vi "ESW (SubVI).vi"(9 "ASW(ZN)":dbl[](array[numeric]), 10 "ASW(KN)":dbl[](array[numeric]), 11 "ESW(in)":dbl[](array[numeric])) -> (3 "ESW(out)":dbl[](array[numeric]))   [LabVIEW 2019]
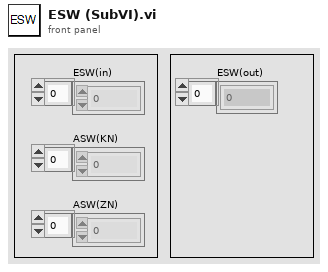
[diagram p1: front panel]
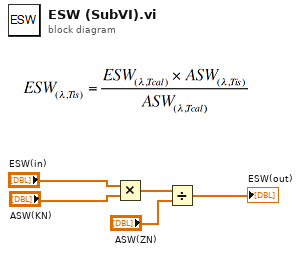
[diagram p0: block diagram]
diagram:
  n1 = Multiply(x="ESW(in)", y="ASW(KN)") -> (x*y=w1:dbl[])
  n2 = Divide(x=w1, y="ASW(ZN)") -> (x/y=→"ESW(out)":dbl[])
